vi "CTRE_CANifier_SetGeneralOutput.vi"(0 "CANifierDevRef":T2, 5 "Output Pin":T1, 7 "Pin State":bool, 9 "Enable as Output?":bool, 11 "error in":errorcluster) -> (4 "CANifierDevRef":T2, 15 "error out":errorcluster)   [LabVIEW 2020]
doc: "Configures a single pin output."
uses:
  <vilib>/Rock Robotics/WPI/ThirdParty/Phoenix-LabVIEW/CANifier/CTRE_CANifier_DeviceRef.ctl
  <vilib>/Rock Robotics/WPI/ThirdParty/Phoenix-LabVIEW/CANifier/CTRE_CANifier_GeneralPin.ctl
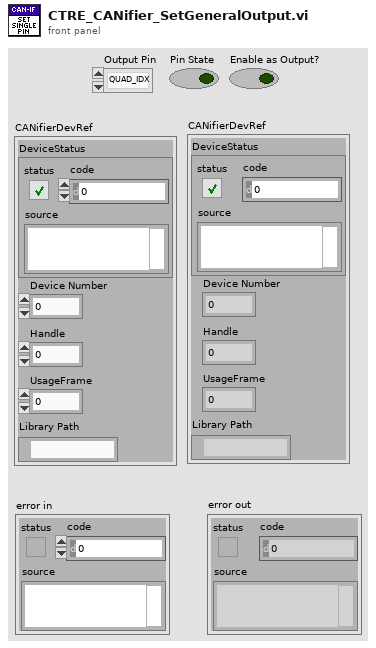
[diagram p1: front panel]
types:
  T1 = typedef "CTRE_CANifier_GeneralPin.ctl" = enum16{"QUAD_IDX", "QUAD_B", "QUAD_A", "LIMR", "LIMF", "SDA", "SCL", "SPI_CS", "SPI_MISO_PWM2", "SPI_MOSI_PWM1", "SPI_CLK_PWM0"}
  T2 = typedef "CTRE_CANifier_DeviceRef.ctl" = cluster{"DeviceStatus":errorcluster, "Device Number":u8, "Handle":u64, "UsageFrame":u32, "Library Path":path}
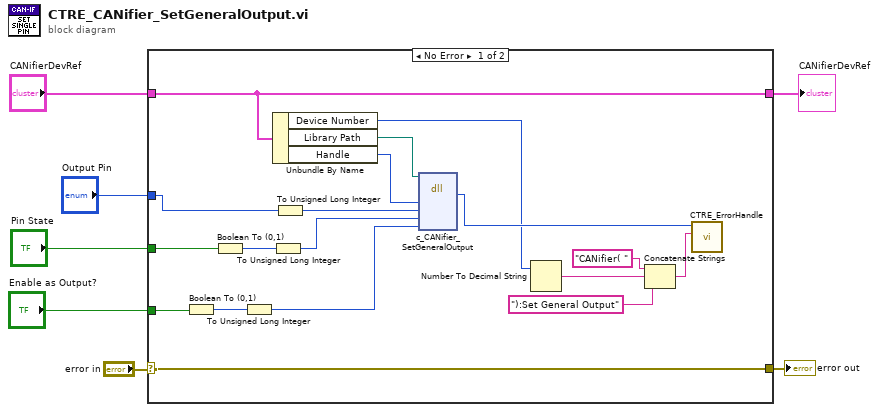
[diagram p0: block diagram]
diagram:
  n1 = case shown="No Error" "error in" {
    selector: "error in" -> [w25 w27]
    tunnel: [w25 w27] -> w6
    tunnel: "CANifierDevRef" -> [w24 w26]
    tunnel: [w24 w26] -> w4
    tunnel: "Output Pin" -> [w15 _]
    tunnel: "Pin State" -> [w13 _]
    tunnel: "Enable as Output?" -> [w9 _]
    frame No Error {
      n2 = Boolean To (0,1)(Boolean=w9) -> (0, 1=w10:i16)
      n3 = Boolean To (0,1)(Boolean=w13) -> (0, 1=w12:i16)
      n4 = To Unsigned Long Integer(number=w10) -> (unsigned 32bit integer=w8:u32)
      n5 = Unbundle By Name(w24) -> ("Device Number"=w17:u8, "Library Path"=w23:path, "Handle"=w22:u64)
      n6 = To Unsigned Long Integer(number=w12) -> (unsigned 32bit integer=w11:u32)
      n7 = To Unsigned Long Integer(number=w15) -> (unsigned 32bit integer=w14:u32)
      n8 = dll-call lib="?" fn="c_CANifier_SetGeneralOutput"(path in=w23, "handle"=w22, "outputPin"=w14, "outputValue"=w11, "outputEnable"=w8) -> ("CTR_Code"=w21:i8)  [unwired: 6 in, 2 out]
      n9 = Number To Decimal String(number=w17) -> (decimal integer string=w20:string)  [unwired: 1 in]
      n10 = Concatenate Strings("CANifier( " ("string"), w20, "):Set General Output" ("string")) -> (w16:string)
      n11 = call <vilib>:"CTRE_ErrorHandle.vi"("origin"=w16, "code"=w21) -> ()  [unwired: 9 in, 1 out]
    }
    frame Error {
    }
  }
  "error out" <- w6
  "CANifierDevRef" <- w4
